vi "Double Exponential Decay.vi"(3 "output control":T1, 4 "data":variant, 5 "X":dbl[](array[numeric]), 6 "a":dbl[](array[numeric])) -> (0 "error out":errorcluster, 1 "f'(X,a)":dbl[][](array[numeric]), 2 "f(X,a)":dbl[](array[numeric]))   [LabVIEW 2022 SP3]
doc: "Implements an ellipse model function to be passed to the Nonlinear Curve Fit.vi."
uses:
  <vilib>/gmath/NumericalOptimization/LM_output select.ctl
  <vilib>/gmath/NI_Gmath.lvlib
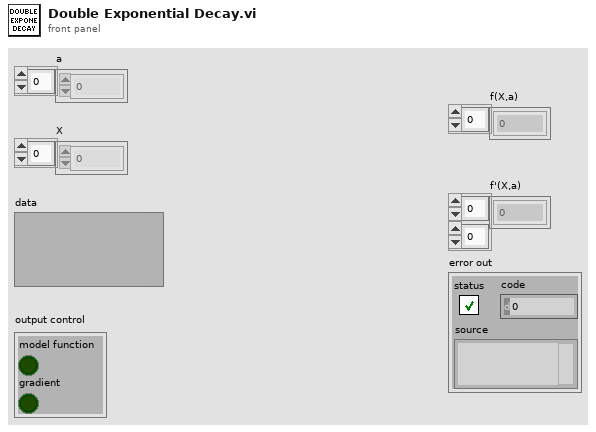
[diagram p1: front panel]
types:
  T1 = typedef "NI_Gmath.lvlib/LM_output select.ctl" = cluster{"model function":bool, "gradient":bool}
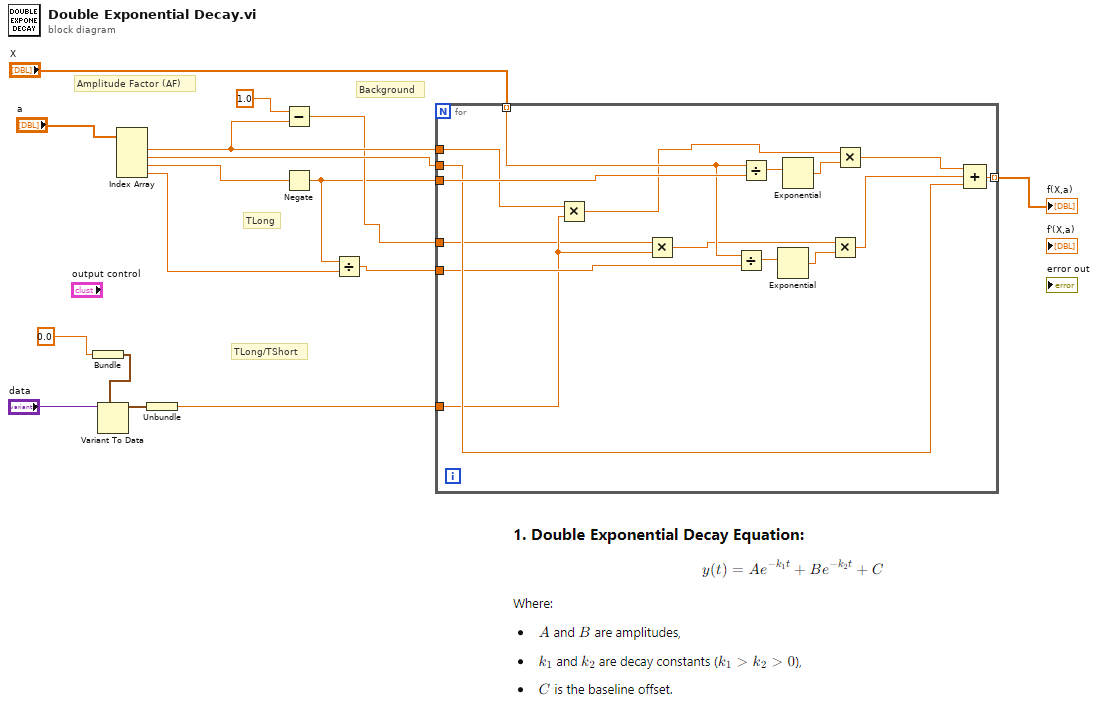
[diagram p0: block diagram]
diagram:
  # "TLong/TShort"
  # "TLong"
  # "Background"
  # "Amplitude Factor (AF)"
  n1 = Bundle(0.0) -> (w11:cluster{dbl})  [unwired: 1 in]
  n2 = Variant To Data(type=w11, Variant="data") -> (data=w10:cluster{dbl})  [unwired: 1 in, 1 out]
  n3 = Index Array(array="a") -> (element #1=w6:dbl, element #2=w9:dbl, element #3=w8:dbl, element #4=w2:dbl)  [unwired: 4 in]
  n4 = Unbundle(w10) -> (w7:dbl)
  n5 = Subtract(x=1.0, y=w6) -> (x-y=w4:dbl)
  n6 = Negate(x=w8) -> (-x=w3:dbl)
  n7 = Divide(x=w3, y=w2) -> (x/y=w1:dbl)
  n8 = for {
    tunnel: w6 -> [w21]
    tunnel: w9 -> [w30]
    tunnel: [w22] -> w15 mode=indexing
    tunnel: "X" -> [w26] mode=indexing
    tunnel: w3 -> [w31]
    tunnel: w1 -> [w25]
    tunnel: w7 -> [w19]
    tunnel: w4 -> [w18]
    n9 = Multiply(x=w21, y=w19) -> (x*y=w20:dbl)
    n10 = Multiply(x=w18, y=w19) -> (x*y=w17:dbl)
    n11 = Divide(x=w26, y=w25) -> (x/y=w27:dbl)
    n12 = Divide(x=w26, y=w31) -> (x/y=w32:dbl)
    n13 = Exponential(1:w27) -> (0:w28:dbl)
    n14 = Exponential(1:w32) -> (0:w29:dbl)
    n15 = Multiply(x=w17, y=w28) -> (x*y=w24:dbl)
    n16 = Multiply(x=w20, y=w29) -> (x*y=w23:dbl)
    n17 = Compound Arithmetic op=ADD(w23, w24, w30) -> (w22:dbl)
  }
  "f(X,a)" <- w15
